vi "Port to Read.vi"(8 "error in (no error)":errorcluster, 10 "Port to Read":dbl, 11 "TI in":refnum<class "TI.lvclass">) -> (0 "error out":errorcluster, 3 "TI out":refnum<class "TI.lvclass">)   [LabVIEW 2020, in "TI.lvclass"]
doc: "Port to read es el vi donde se manda al microcontrolador los datos del puerto que se desea leer"
uses:
  TI.lvclass
  TI.lvclass/TI.ctl
  feb8519b-fa08-48e8-9854-c43e3d7b396b.vi
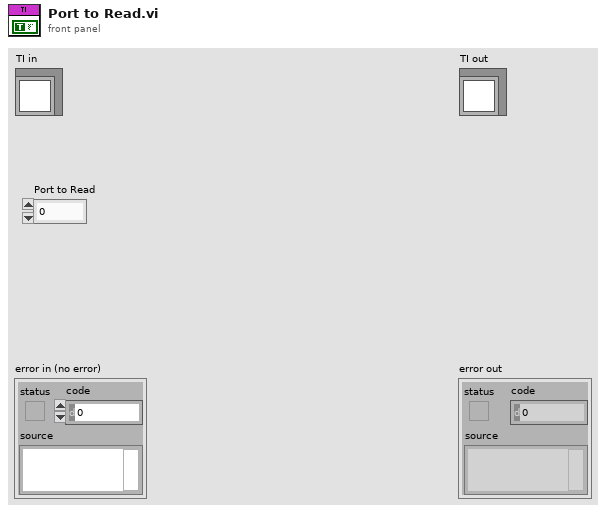
[diagram p1: front panel]
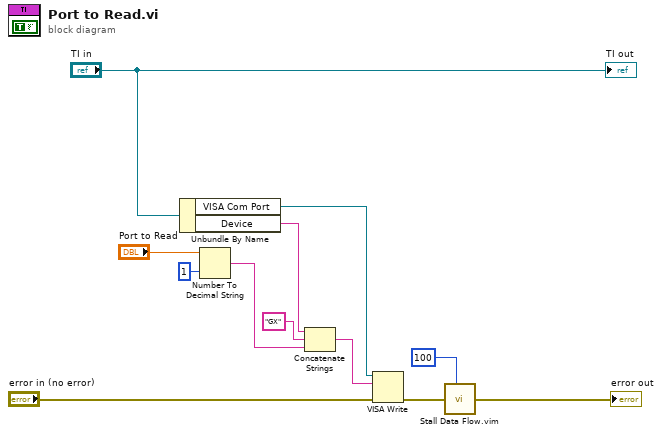
[diagram p0: block diagram]
diagram:
  n1 = Unbundle By Name("TI in") -> ("VISA Com Port"=w11:refnum<visa-resource-name>, "Device"=w9:string)
  n2 = Number To Decimal String(number="Port to Read", width (-)=i16 1) -> (decimal integer string=w8:string)
  n3 = Concatenate Strings(w9, "GX" ("string"), w8) -> (w10:string)
  n4 = VISA Write(VISA resource name=w11, write buffer=w10, error in (no error)="error in (no error)") -> (error out=w12:errorcluster)  [unwired: 2 out]
  n5 = call "Stall Data Flow.vim"("value in"=w12, "milliseconds to wait"=u32 100) -> ("value out"=→"error out":errorcluster)  [unwired: 1 out]
  "TI out" <- "TI in"
